vi "3rd.vi"   [LabVIEW 2016]
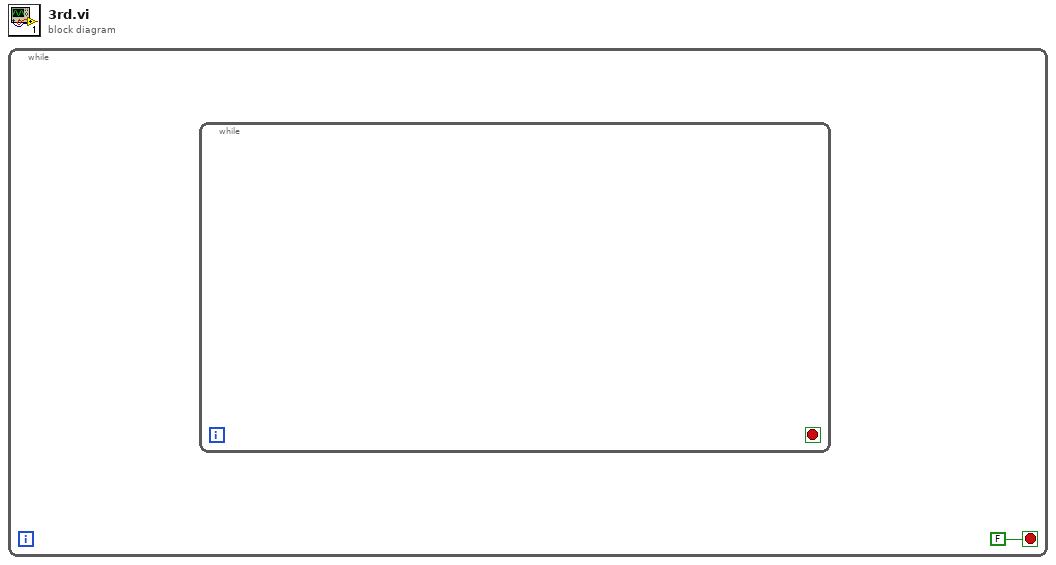
[diagram p0: block diagram]
diagram:
  n1 = while {
    stop <- FALSE stop-if-true
    n2 = while {
      stop <- _ stop-if-true
    }
  }
